vi "DeleteWhitespace.vi"(0 "string":string caption="字符串", 1 "location (both)":T1 caption="位置（两端）" items=["两端", "字符串首端", "字符串末端"]) -> (2 "trimmed string":string caption="删减后字符串")   [LabVIEW 2011]
doc: "在<B>字符串</B>的起始、末尾或两端删除所有空白（空格、制表符、回车符和换行符）。该VI不删除双字节字符。"
uses:
  <vilib>/Utility/error.llb/whitespace.ctl
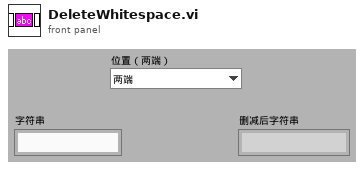
[diagram p1: front panel]
types:
  T1 = typedef "whitespace.ctl" = u16
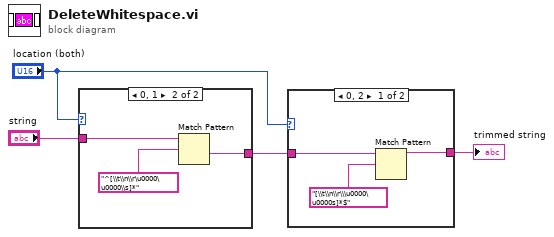
[diagram p0: block diagram]
diagram:
  n1 = case shown="0, 1" "location (both)" {
    tunnel: [w5 w8] -> w3
    tunnel: "string" -> [w5 w6]
    frame Default {
    }
    frame 0, 1 {
      n2 = Match Pattern(string=w6, regular expression="^[\\t\\n\\r\u0000\u0000\\s]*") -> (after substring=w8:string)  [unwired: 1 in, 3 out]
    }
  }
  n3 = case shown="0, 2" "location (both)" {
    tunnel: [w11 w12] -> w4
    tunnel: w3 -> [w10 w12]
    frame 0, 2 {
      n4 = Match Pattern(string=w10, regular expression="[\\t\\n\\r\\\u0000\u0000s]*$") -> (before substring=w11:string)  [unwired: 1 in, 3 out]
    }
    frame Default {
    }
  }
  "trimmed string" <- w4
